vi "Cuboid initial preprocessing.vi"(1 "Cuboid properties in":T1={"Vertices (x, y)"=[[0.0, 0.0, 0.0], [1.0, 1.0, 0.0], [0.0, 1.0, 0.0], [1.0, 0.0, 0.0]], "Zmin"=0.0, "Zmax"=1.0, "Centroid (x, y)"=[0.0, 0.0, 0.0], "Radius"=0.0, "Edge normals (x, y)"=[[0.0, 0.0, 0.0], [0.0, 0.0, 0.0], [0.0, 0.0, 0.0], [0.0, 0.0, 0.0]], "Edge vectors (x, y)"=[[0.0, 0.0], [0.0, 0.0], [0.0, 0.0], [0.0, 0.0]]}) -> (0 "Cuboid properties out":T1={"Vertices (x, y)"=[[1.0, 0.0], [1.0, 1.0], [0.0, 1.0], [0.0, 0.0]], "Zmin"=0.0, "Zmax"=1.0, "Centroid (x, y)"=[0.5, 0.5, 0.0], "Radius"=0.7071067811865476, "Edge normals (x, y)"=[[1.0, 0.0], [0.0, 1.0], [-1.0, 0.0], [0.0, -1.0]], "Edge vectors (x, y)"=[[0.0, 1.0], [-1.0, 0.0], [0.0, -1.0], [1.0, 0.0]]})   [LabVIEW 2014]
uses:
  Cuboids sub vis/Cuboid properties.ctl
  <vilib>/Analysis/baseanly.llb/Real Dot Product.vi
  <vilib>/Analysis/_algsub.llb/Real Vector Norm.vi
  <vilib>/Analysis/baseanly.llb/Unit Vector (DBL).vi
  <vilib>/Analysis/NI_AALBase.lvlib
  <vilib>/Analysis/NI_AALPro.lvlib
panel:
  # "Initial preprocessing ensures the vertices are wound anticlockwise. This only needs to be done once. Subsequent transformations of the vertices need only pass through the standard preprocessing sub vi."
  # "PN 30/08/2014"
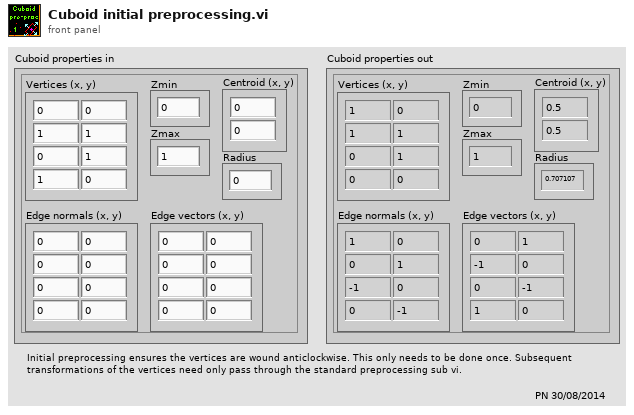
[diagram p1: front panel]
types:
  T1 = typedef "Cuboid properties.ctl" = cluster{"Vertices (x, y)":dbl[][], "Zmin":dbl, "Zmax":dbl, "Centroid (x, y)":dbl[], "Radius":dbl, "Edge normals (x, y)":dbl[][], "Edge vectors (x, y)":dbl[][]}
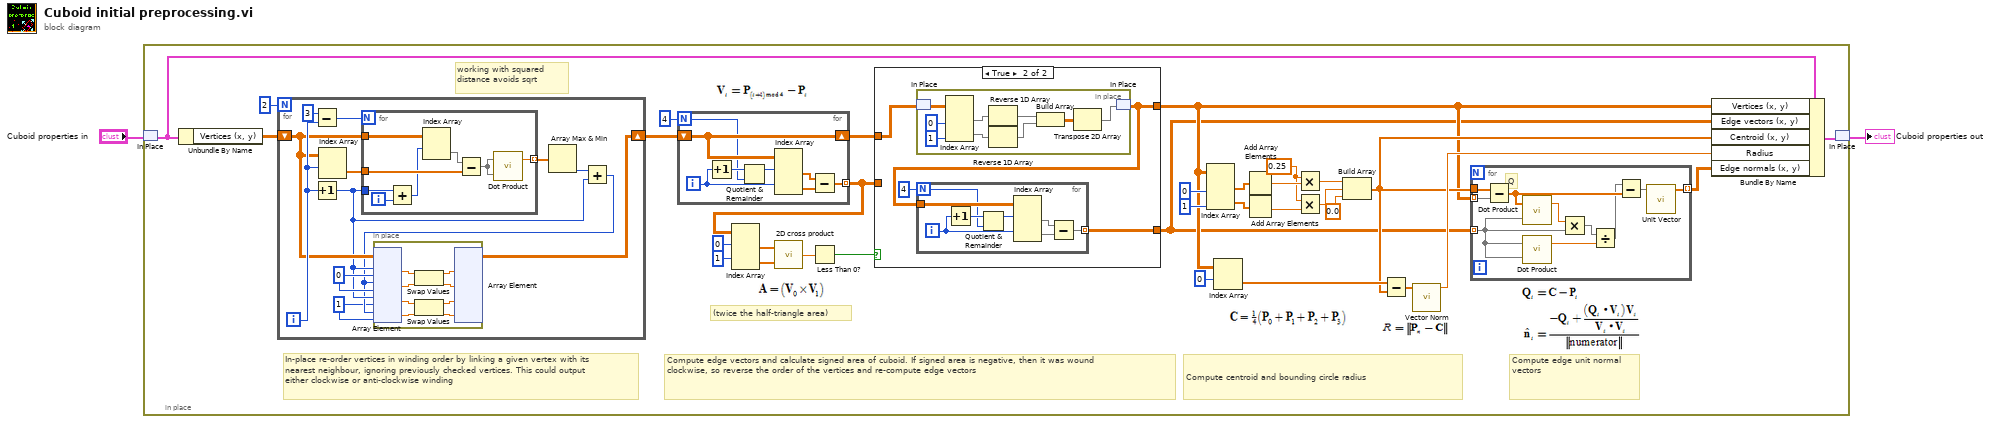
[diagram p0: block diagram]
diagram:
  n1 = in-place {
    w20 = 0.25 ("x")
    # "Compute edge unit normal vectors"
    # "working with squared distance avoids sqrt"
    # "(twice the half-triangle area)"
    # "Compute centroid and bounding circle radius"
    # "Compute edge vectors and calculate signed area of cuboid. If signed area is negative, then it was wound clockwise, so reverse the order of the vertices and re-compute edge vectors"
    # "In-place re-order vertices in winding order by linking a given vertex with its nearest neighbour, ignoring previously checked vertices. This could output either clockwise or anti-clockwise winding"
    n2 = in-place-match #1("Cuboid properties in") -> (w12:T1)
    n3 = Unbundle By Name(w12) -> ("Vertices (x, y)"=w34:dbl[][])
    n4 = for {
      N: 2 -> [_]
      shift-right: [w76] -> w32
      shift-left: w34 -> [w84]
      i -> [w85]
      w77 = 1
      w83 = 0
      n5 = Subtract(x=3, y=w85) -> (x-y=w80:i32)
      n6 = Increment(x=w85) -> (x+1=w79:i32)
      n7 = Index Array(array=w84, index (row)=w85) -> (element=w87:dbl[])  [unwired: 1 in]
      n8 = for {
        N: w80 -> [_]
        tunnel: w87 -> [w99]
        tunnel: w84 -> [w101]
        tunnel: w79 -> [w102]
        tunnel: [w97] -> w86 mode=indexing
        i -> [w103]
        n9 = Add(x=w102, y=w103) -> (x+y=w96:i32)
        n10 = Index Array(array=w101, index (row)=w96) -> (element=w100:dbl[])  [unwired: 1 in]
        n11 = Subtract(x=w100, y=w99) -> (x-y=w98:dbl[])
        n12 = call-poly <vilib>:"Dot Product.vi"("Y Vector"=w98, "X Vector"=w98) -> ("X * Y"=w97:dbl)  [unwired: 1 out]
      }
      n13 = Array Max & Min(array=w86) -> (min index (indices)=w82:i32)  [unwired: 3 out]
      n14 = Add(x=w82, y=w79) -> (x+y=w78:i32)
      n15 = in-place {
        n16 = in-place-array #2(w84, w79, w83, w78, w83, w79, w77, w78, w77) -> (w95:dbl, w94:dbl, w91:dbl, w90:dbl)
        n17 = Swap Values(12:w95, 14:w94) -> (1:w93:dbl, 3:w92:dbl)  [unwired: 1 in]
        n18 = Swap Values(12:w91, 14:w90) -> (1:w89:dbl, 3:w88:dbl)  [unwired: 1 in]
        n19 = in-place-array #2(w93, w92, w89, w88) -> (w76:dbl[][])  [unwired: 8 out]
      }
    }
    n20 = for {
      N: 4 -> [w69]
      shift-right: [w75] -> w27
      shift-left: w32 -> [w75]
      tunnel: [w71] -> w11 mode=indexing
      i -> [w74]
      n21 = Increment(x=w74) -> (x+1=w70:i32)
      n22 = Quotient & Remainder(x=w70, y=w69) -> (x-y*floor(x/y)=w68:i32)  [unwired: 1 out]
      n23 = Index Array(array=w75, index (row) #1=w68, index (row) #2=w74) -> (element #1=w73:dbl[], element #2=w72:dbl[])  [unwired: 2 in]
      n24 = Subtract(x=w73, y=w72) -> (x-y=w71:dbl[])
    }
    n25 = Index Array(array=w11, index (row) #1=0 ("index (row)"), index (row) #2=1 ("index (row)")) -> (element #1=w10:dbl[], element #2=w9:dbl[])  [unwired: 2 in]
    n26 = call "2D cross product.vi"("B"=w9, "A"=w10) -> ("A X B"=w8:dbl)
    n27 = Less Than 0?(x=w8) -> (x < 0?=w28:bool)
    n28 = case shown="True" w28 {
      tunnel: [w45 w47] -> w4
      tunnel: w27 -> [w46 w50]
      tunnel: [w46 w48] -> w6
      tunnel: w11 -> [w45 _]
      frame False {
        # "already wound anti-clockwise, just continue"
      }
      frame True {
        n29 = in-place {
          n30 = in-place-match #3(w50) -> (w67:dbl[][])
          n31 = Index Array(array=w67, index (col) #1=0 ("disabled index (col)"), index (col) #2=1 ("index (col)")) -> (element #1=w64:dbl[], element #2=w63:dbl[])  [unwired: 2 in]
          n32 = Reverse 1D Array(array=w64) -> (reversed array=w62:dbl[])
          n33 = Reverse 1D Array(array=w63) -> (reversed array=w61:dbl[])
          n34 = Build Array(w62, w61) -> (w60:dbl[][])
          n35 = Transpose 2D Array(2D array=w60) -> (transposed array=w59:dbl[][])
          n36 = in-place-match #3(w59) -> (w48:dbl[][])
        }
        n37 = for {
          N: 4 -> [w52]
          tunnel: [w54] -> w47 mode=indexing
          tunnel: w48 -> [w58]
          i -> [w57]
          n38 = Increment(x=w57) -> (x+1=w53:i32)
          n39 = Quotient & Remainder(x=w53, y=w52) -> (x-y*floor(x/y)=w51:i32)  [unwired: 1 out]
          n40 = Index Array(array=w58, index (row) #1=w51, index (row) #2=w57) -> (element #1=w56:dbl[], element #2=w55:dbl[])  [unwired: 2 in]
          n41 = Subtract(x=w56, y=w55) -> (x-y=w54:dbl[])
        }
      }
    }
    n42 = Index Array(array=w6, index (col) #1=0 ("disabled index (col)"), index (col) #2=1 ("index (col)")) -> (element #1=w24:dbl[], element #2=w23:dbl[])  [unwired: 2 in]
    n43 = Index Array(array=w6, index (row)=0) -> (element=w15:dbl[])  [unwired: 1 in]
    n44 = Add Array Elements(numeric array=w24) -> (sum=w22:dbl)
    n45 = Add Array Elements(numeric array=w23) -> (sum=w21:dbl)
    n46 = Multiply(x=w20, y=w22) -> (x*y=w19:dbl)
    n47 = Multiply(x=w20, y=w21) -> (x*y=w18:dbl)
    n48 = Build Array(w19, w18, 0.0 ("element")) -> (w7:dbl[])
    n49 = Subtract(x=w15, y=w7) -> (x-y=w14:dbl[])
    n50 = call-poly <vilib>:"Vector Norm.vi"("Input Vector"=w14) -> ("norm"=w13:dbl)  [unwired: 9 in, 1 out]
    n51 = for {
      tunnel: [w44] -> w5 mode=indexing
      tunnel: w4 -> [w39] mode=indexing
      tunnel: w7 -> [w43]
      tunnel: w6 -> [w42] mode=indexing
      # "Q"
      n52 = Subtract(x=w43, y=w42) -> (x-y=w41:dbl[])
      n53 = call-poly <vilib>:"Dot Product.vi"("Y Vector"=w39, "X Vector"=w41) -> ("X * Y"=w40:dbl)  [unwired: 1 out]
      n54 = call-poly <vilib>:"Dot Product.vi"("Y Vector"=w39, "X Vector"=w39) -> ("X * Y"=w38:dbl)  [unwired: 1 out]
      n55 = Multiply(x=w40, y=w39) -> (x*y=w37:dbl[])
      n56 = Divide(x=w37, y=w38) -> (x/y=w36:dbl[])
      n57 = Subtract(x=w36, y=w41) -> (x-y=w35:dbl[])
      n58 = call-poly <vilib>:"Unit Vector.vi"("Input Vector"=w35) -> ("Unit Vector"=w44:dbl[])  [unwired: 8 in, 2 out]
    }
    n59 = Bundle By Name(cluster=w12, "Vertices (x, y)"=w6, "Edge vectors (x, y)"=w4, "Centroid (x, y)"=w7, "Radius"=w13, "Edge normals (x, y)"=w5) -> (w3:T1)
    n60 = in-place-match #1(w3) -> (→"Cuboid properties out":T1)
  }
